vi "mecanum.vi"(9 "rx":dbl, 10 "X":dbl, 11 "Y":dbl) -> (0 "BR":dbl, 1 "FR":dbl, 2 "BL":dbl, 3 "FL":dbl)   [LabVIEW 2019]
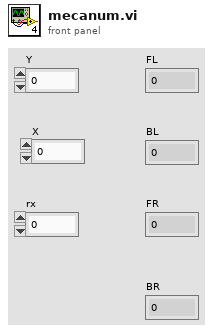
[diagram p1: front panel]
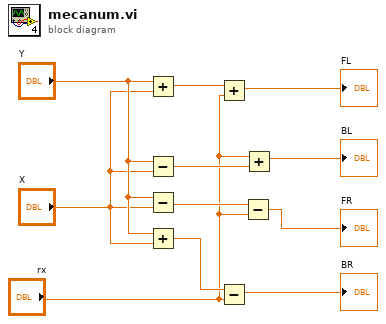
[diagram p0: block diagram]
diagram:
  n1 = Add(x="Y", y="X") -> (x+y=w1:dbl)
  n2 = Subtract(x="Y", y="X") -> (x-y=w10:dbl)
  n3 = Subtract(x="Y", y="X") -> (x-y=w8:dbl)
  n4 = Add(x="Y", y="X") -> (x+y=w6:dbl)
  n5 = Add(x=w1, y="rx") -> (x+y=→"FL":dbl)
  n6 = Subtract(x=w6, y="rx") -> (x-y=→"BR":dbl)
  n7 = Subtract(x=w8, y="rx") -> (x-y=→"FR":dbl)
  n8 = Add(x="rx", y=w10) -> (x+y=→"BL":dbl)
